vi "Read Sim Speed.vi"(8 "error in (no error)":errorcluster, 11 "Pump.Simulated in":refnum<class "Pump.Simulated.lvclass">) -> (0 "error out":errorcluster, 2 "Sim Speed":refnum<data-value>, 3 "Pump.Simulated out":refnum<class "Pump.Simulated.lvclass">)   [LabVIEW 2014, in "Pump.Simulated.lvclass"]
uses:
  Pump.Simulated.lvclass
  Pump.Simulated.lvclass/Pump.Simulated.ctl
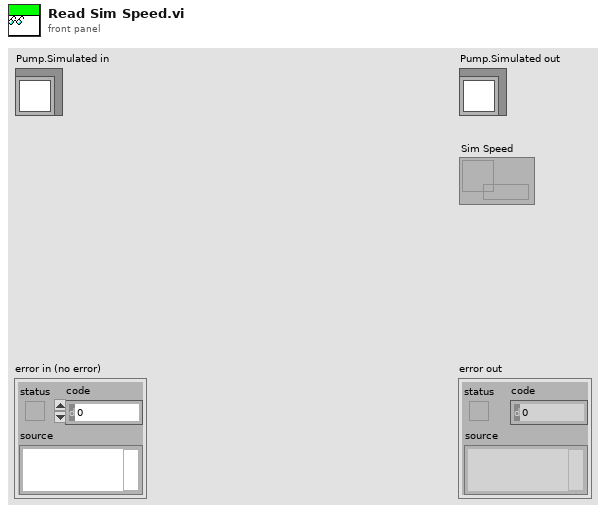
[diagram p1: front panel]
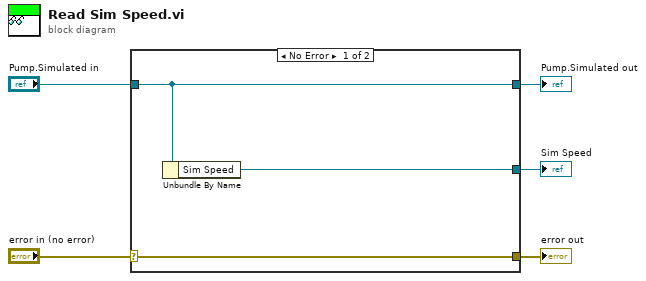
[diagram p0: block diagram]
diagram:
  n1 = case shown="No Error" "error in (no error)" {
    selector: "error in (no error)" -> [w8 w9]
    tunnel: [w8 w9] -> w4
    tunnel: [w7 w10] -> w2
    tunnel: "Pump.Simulated in" -> [w7 w10]
    tunnel: [w6 _] -> w1
    frame No Error {
      n2 = Unbundle By Name(w7) -> ("Sim Speed"=w6:refnum<data-value>)
    }
    frame Error {
    }
  }
  "error out" <- w4
  "Pump.Simulated out" <- w2
  "Sim Speed" <- w1
